vi "Serienschaltung.vi"(2 "error in (no error)":errorcluster, 3 "Array In":dbl[](array[numeric])) -> (0 "error out":errorcluster, 1 "Out":dbl)   [LabVIEW 2022 SP3]
uses:
  <vilib>/Utility/error.llb/Error Cluster From Error Code.vi
  <vilib>/ErrorRing/Error Ring.xnode
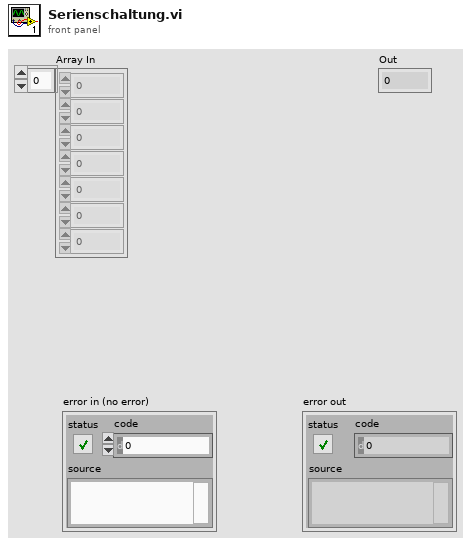
[diagram p1: front panel]
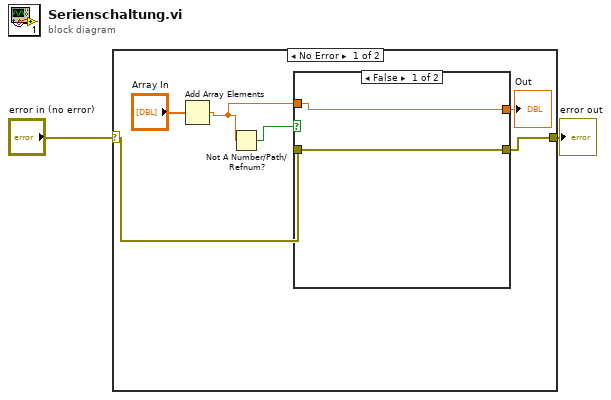
[diagram p0: block diagram]
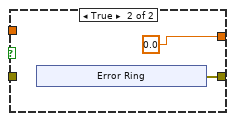
[diagram p2: hidden frame]
diagram:
  n1 = case shown="No Error" "error in (no error)" {
    selector: "error in (no error)" -> [w7 w18]
    tunnel: [w6 w18] -> w1
    frame No Error {
      n2 = Add Array Elements(numeric array="Array In") -> (sum=w3:dbl)
      n3 = Not A Number/Path/Refnum?(number/path/refnum=w3) -> (NaN/Path/Refnum?=w4:bool)
      n4 = case shown="False" w4 {
        tunnel: [w10 w12] -> w6
        tunnel: w7 -> [w10 _]
        tunnel: w3 -> [w9 _]
        tunnel: [w9 0.0] -> w5
        frame False {
        }
        frame True {
          n5 = xnode "Error Ring"() -> ("error out"=w12:errorcluster)
        }
      }
      "Out" <- w5
    }
    frame Error {
    }
  }
  "error out" <- w1
